vi "InstrChoice.vi"(0 "Instrument IN":string, 3 "SkipChoixInstr":bool, 5 "instruments.ini":path, 7 "DisallowUndo":bool) -> (10 "This VI's Path":path, 13 "Modifier?":bool, 14 "Instrument OUT":string, 15 "FoV":dbl caption="Champ de Vue" format="%.2g", 16 "foynom":i32 caption="Foyer nominale à 0°", 17 "atherm":dbl caption="Coefficient d'athermalisation" format="%.3g", 18 "exclusion":path caption="Chemin vers le fichier d'exclusion", 19 "collim":path caption="Chemin vers le fichier de collimation")   [LabVIEW 2019]
uses:
  <vilib>/Utility/config.llb/Read Key (Double).vi
  <vilib>/Utility/config.llb/Read Key (I32).vi
  <vilib>/Utility/config.llb/Read Key (Path).vi
  <vilib>/Utility/config.llb/NI_LVConfig.lvlib
panel:
  in  "cancel":bool
  in  "ok":bool
  in  "Instruments":i32(ring) items=["Pesto", "Cpapir", "Simon", "Spectro", "SpiOMM", "PANO-II+CCD4Kx4K", "CCD4Kx4K", "PANO-I+EMCCD", "POLARIMETRE"]
  # "[minutes d'arc]"
  # "[ADU]"
  # "[ADU/°K]"
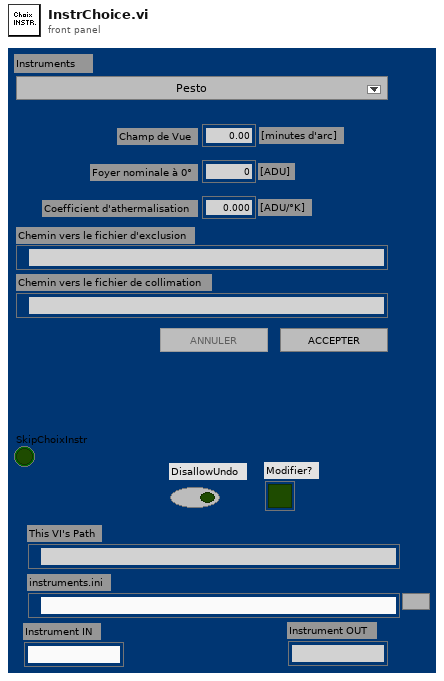
[diagram p1: front panel]
types:
  T1 = typedef "NI_LVConfig.lvlib/Config Data RefNum.ctl" = refnum<k1>
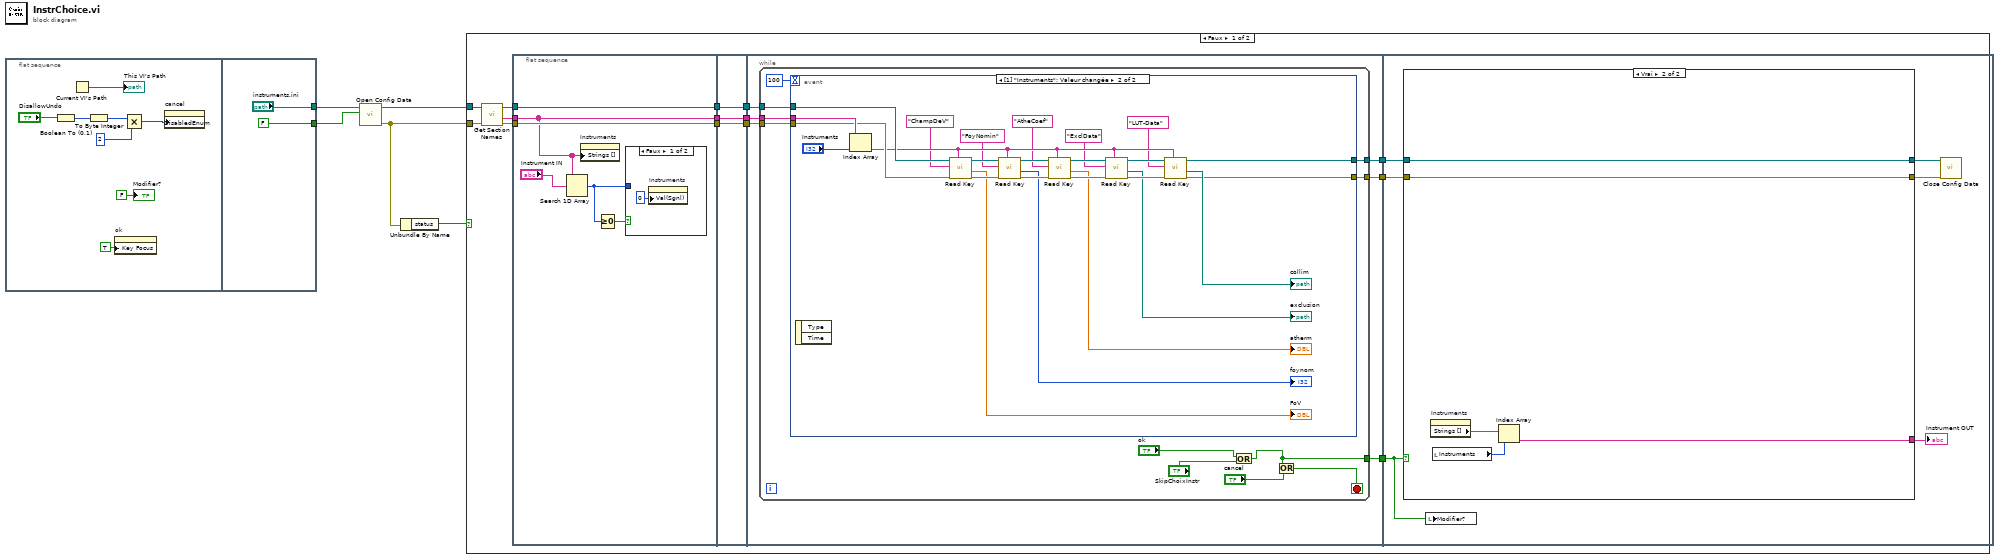
[diagram p0: block diagram]
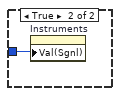
[diagram p2: hidden frame]
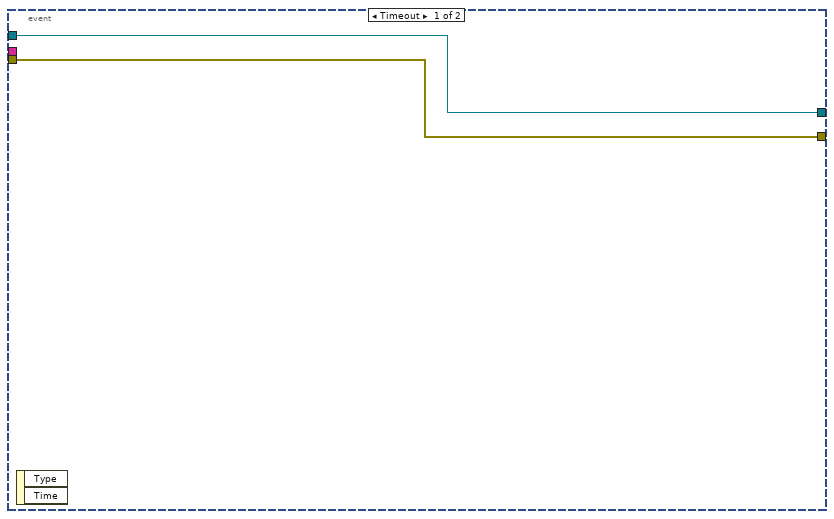
[diagram p3: hidden frame]
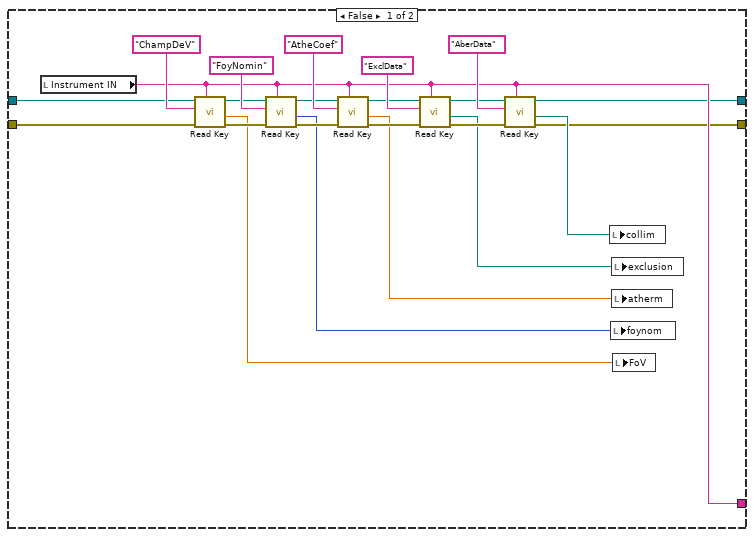
[diagram p4: hidden frame]
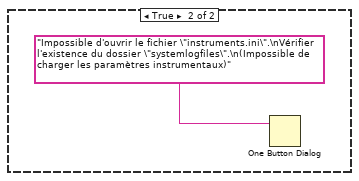
[diagram p5: hidden frame]
diagram:
  n1 = flat-sequence {
    tunnel: [FALSE ("create file if necessary (T)")] -> w5
    tunnel: ["instruments.ini"] -> w1
    frame #0 {
      n2 = Boolean To (0,1)(Boolean="DisallowUndo") -> (0, 1=w12:i16)
      n3 = Current VI's Path() -> (path=→"This VI's Path":path)
      n4 = To Byte Integer(number=w12) -> (8bit integer=w10:i8)
      n5 = property on="ok" class="Bool"("Key Focus"=TRUE) -> ()  [unwired: 2 in, 2 out]
      n6 = Multiply(x=w10, y=i8 2) -> (x*y=w9:i8)
      n7 = property on="cancel" class="Bool"("DisabledEnum"=w9) -> ()  [unwired: 2 in, 2 out]
      "Modifier?" <- FALSE ("Modifier?")
    }
    frame #1 {
    }
  }
  n8 = call <vilib>:"Open Config Data.vi"("create file if necessary (T)"=w5, "configuration file path"=w1) -> ("error out"=w3:errorcluster, "refnum"=w4:T1)  [unwired: 7 in, 1 out]
  n9 = Unbundle By Name(w3) -> ("status"=w2:bool)
  n10 = case shown="Faux" w2 {
    tunnel: w4 -> [w29 _]
    tunnel: w3 -> [w28 _]
    frame False {
      n11 = call <vilib>:"Get Section Names.vi"("error in (no error)"=w28, "refnum"=w29) -> ("error out"=w25:errorcluster, "section names"=w26:string[], "refnum out"=w27:T1)  [unwired: 7 in]
      n12 = flat-sequence {
        tunnel: w27 -> [w34]
        tunnel: w26 -> [w30]
        tunnel: [w35] -> w21
        tunnel: w25 -> [w35]
        tunnel: [w34] -> w19
        tunnel: [w30] -> w17
        tunnel: w21 -> [w40]
        tunnel: [w40] -> w20
        tunnel: w19 -> [w39]
        tunnel: [w39] -> w18
        tunnel: w17 -> [w38]
        tunnel: [w38] -> w16
        tunnel: w20 -> [w44]
        tunnel: w18 -> [w45]
        tunnel: w16 -> [w46]
        tunnel: [w43] -> w24
        tunnel: [w42] -> w23
        tunnel: [w41] -> w22
        tunnel: w24 -> [w85]
        tunnel: w23 -> [w89]
        tunnel: w22 -> [w88]
        frame #0 {
          n13 = Search 1D Array(1D array=w30, element="Instrument IN") -> (index of element=w31:i32)  [unwired: 1 in]
          n14 = property on="Instruments" class="MDér (strict)"("Strings []"=w30) -> ()  [unwired: 2 in, 2 out]
          n15 = Greater Or Equal To 0?(x=w31) -> (x >= 0?=w32:bool)
          n16 = case shown="Faux" w32 {
            tunnel: w31 -> [_ w37]
            frame False {
              n17 = property on="Instruments" class="MDér (strict)"("Val(Sgnl)"=0) -> ()  [unwired: 2 in, 2 out]
            }
            frame True {
              n18 = property on="Instruments" class="MDér (strict)"("Val(Sgnl)"=w37) -> ()  [unwired: 2 in, 2 out]
            }
          }
        }
        frame #1 {
        }
        frame #2 {
          n19 = while {
            tunnel: w46 -> [w57]
            tunnel: w45 -> [w56]
            tunnel: w44 -> [w55]
            tunnel: [w47] -> w43
            tunnel: [w51] -> w42
            tunnel: [w50] -> w41
            stop <- w52 stop-if-true
            n20 = event shown="[1] \"Instruments\": Valeur changée" {
              selector: _ -> [_ _]
              dyn-events: _ -> [_ _]
              timeout: 100 ("milliseconds to wait") -> [_ _]
              tunnel: w57 -> [_ w83]
              tunnel: w56 -> [w59 w82]
              tunnel: w55 -> [w58 w81]
              tunnel: [w59 w61] -> w51
              tunnel: [w58 w60] -> w50
              event Timeout {
                n21 = event-data() -> ()  [unwired: 1 in, 2 out]
              }
              event "Instruments": Value Change {
                n22 = event-data() -> ()  [unwired: 1 in, 2 out]
                n23 = Index Array(array=w83, index="Instruments") -> (element=w72:string)
                n24 = call-poly <vilib>:"Read Key.vi"("section"=w72, "error in (no error)"=w81, "key"="ChampDeV", "refnum"=w82) -> ("error out"=w79:errorcluster, "value"=→"FoV":dbl, "refnum out"=w80:T1)  [unwired: 4 in, 1 out]
                n25 = call-poly <vilib>:"Read Key.vi"("section"=w72, "error in (no error)"=w79, "key"="FoyNomin", "refnum"=w80) -> ("error out"=w77:errorcluster, "value"=→"foynom":i32, "refnum out"=w78:T1)  [unwired: 4 in, 1 out]
                n26 = call-poly <vilib>:"Read Key.vi"("section"=w72, "error in (no error)"=w77, "key"="AtheCoef", "refnum"=w78) -> ("error out"=w73:errorcluster, "value"=→"atherm":dbl, "refnum out"=w74:T1)  [unwired: 4 in, 1 out]
                n27 = call-poly <vilib>:"Read Key.vi"("section"=w72, "error in (no error)"=w73, "key"="ExclData", "refnum"=w74) -> ("error out"=w76:errorcluster, "value"=→"exclusion":path, "refnum out"=w75:T1)  [unwired: 4 in, 1 out]
                n28 = call-poly <vilib>:"Read Key.vi"("section"=w72, "error in (no error)"=w76, "key"="LUT-Data", "refnum"=w75) -> ("error out"=w60:errorcluster, "value"=→"collim":path, "refnum out"=w61:T1)  [unwired: 4 in, 1 out]
              }
            }
            n29 = Or(x="ok", y="SkipChoixInstr") -> (x .or. y?=w47:bool)
            n30 = Or(x=w47, y="cancel") -> (x .or. y?=w52:bool)
          }
        }
        frame #3 {
          n31 = case shown="Vrai" w85 {
            tunnel: [w93 w116] -> w90
            tunnel: w89 -> [w100 w115]
            tunnel: w88 -> [w99 w114]
            tunnel: [w92 w115] -> w87
            tunnel: [w91 w114] -> w86
            frame False {
              n32 = local read "Instrument IN"() -> (w93:string)
              n33 = call-poly <vilib>:"Read Key.vi"("section"=w93, "error in (no error)"=w99, "key"="ChampDeV", "refnum"=w100) -> ("error out"=w102:errorcluster, "value"=w94:dbl, "refnum out"=w101:T1)  [unwired: 4 in, 1 out]
              n34 = call-poly <vilib>:"Read Key.vi"("section"=w93, "error in (no error)"=w102, "key"="FoyNomin", "refnum"=w101) -> ("error out"=w104:errorcluster, "value"=w95:i32, "refnum out"=w103:T1)  [unwired: 4 in, 1 out]
              n35 = call-poly <vilib>:"Read Key.vi"("section"=w93, "error in (no error)"=w104, "key"="AtheCoef", "refnum"=w103) -> ("error out"=w108:errorcluster, "value"=w96:dbl, "refnum out"=w107:T1)  [unwired: 4 in, 1 out]
              n36 = call-poly <vilib>:"Read Key.vi"("section"=w93, "error in (no error)"=w108, "key"="ExclData", "refnum"=w107) -> ("error out"=w105:errorcluster, "value"=w97:path, "refnum out"=w106:T1)  [unwired: 4 in, 1 out]
              n37 = call-poly <vilib>:"Read Key.vi"("section"=w93, "error in (no error)"=w105, "key"="AberData", "refnum"=w106) -> ("error out"=w91:errorcluster, "value"=w98:path, "refnum out"=w92:T1)  [unwired: 4 in, 1 out]
              n38 = local write "collim"(w98) -> ()
              n39 = local write "foynom"(w95) -> ()
              n40 = local write "exclusion"(w97) -> ()
              n41 = local write "atherm"(w96) -> ()
              n42 = local write "FoV"(w94) -> ()
            }
            frame True {
              n43 = property on="Instruments" class="MDér (strict)"() -> ("Strings []"=w117:string[])  [unwired: 2 in, 2 out]
              n44 = local read "Instruments"() -> (w118:i32)
              n45 = Index Array(array=w117, index=w118) -> (element=w116:string)
            }
          }
          "Instrument OUT" <- w90
          n46 = local write "Modifier?"(w85) -> ()
          n47 = call <vilib>:"Close Config Data.vi"("error in (no error)"=w86, "refnum"=w87) -> ()  [unwired: 8 in, 2 out]
        }
      }
    }
    frame True {
      n48 = One Button Dialog(message="Impossible d'ouvrir le fichier \"instruments.ini\".\nVérifier l'existence du dossier \"systemlogfiles\".\n(Impossible de charger les paramètres instrumentaux)") -> ()  [unwired: 1 in, 1 out]
    }
  }
